vi "Replication and Deployment Utility.vi"() -> ()   [LabVIEW 2016]
uses:
  subVIs/TypeDefs/rad_State Data.ctl
  subVIs/Targets/TypeDefs/rad_Targets Settings.ctl
  subVIs/Targets/TypeDefs/rad_Target Information.ctl
  subVIs/Targets/TypeDefs/rad_Target Network Settings.ctl
  subVIs/App Images/TypeDefs/rad_App Images Settings.ctl
  subVIs/App Images/TypeDefs/rad_AppImage Information.ctl
  subVIs/App Images/TypeDefs/rad_Application Image Properties.ctl
  subVIs/App Images/TypeDefs/rad_FPGA Properties.ctl
  subVIs/App Images/TypeDefs/rad_FPGA Flash Properties.ctl
  subVIs/Util/Controls/Exit Button.ctl
  subVIs/Util/Controls/Retrieve Button.ctl
  subVIs/Util/Controls/Refresh Button.ctl
  subVIs/Util/Controls/Configure Button.ctl
  subVIs/Util/Controls/Deploy Button.ctl
  subVIs/Util/Controls/Select All Button.ctl
  subVIs/Util/Controls/Add Target Button.ctl
  subVIs/Util/Controls/Compare Button.ctl
  subVIs/Util/FP Control/FP Control Functions.ctl
  <vilib>/Utility/miscctls.llb/LVRowAndColumnUnsignedTypeDef.ctl
  subVIs/RT Image Compare/TypeDefs/rad_Comparison Modes.ctl
  <vilib>/nisyscfg/Close (System).vi
  subVIs/rad_Globals.vi
  <vilib>/nisyscfg/nisyscfg.lvlib
  <resource>/objmgr/nisysapi.rc
panel:
  in  "Targets Settings":bool
  in  "Refresh Targets":T1
  in  "Target List":i32[](listbox)=[0]
  in  "Add Target":T2
  in  "Select All":T3
  in  "Configure Targets":T4
  in  "Compare":T5
  in  "Deploy":T6
  in  "Retrieve":T7
  in  "State":T8 {"Targets Information"."Primary NIC"."IP Address Request Mode" items=["Static"=1, "DHCP/Link-Local"=2, "Link-Local Only"=4, "DHCP Only"=8]}
  in  "App Images Settings":bool
  in  "Refresh Apps":T1
  in  "Exit":T17
  in  "App Images List":i32(listbox)=6
  in  "Configure App":T4
  # "Deployment Targets"
  # "Application Images"
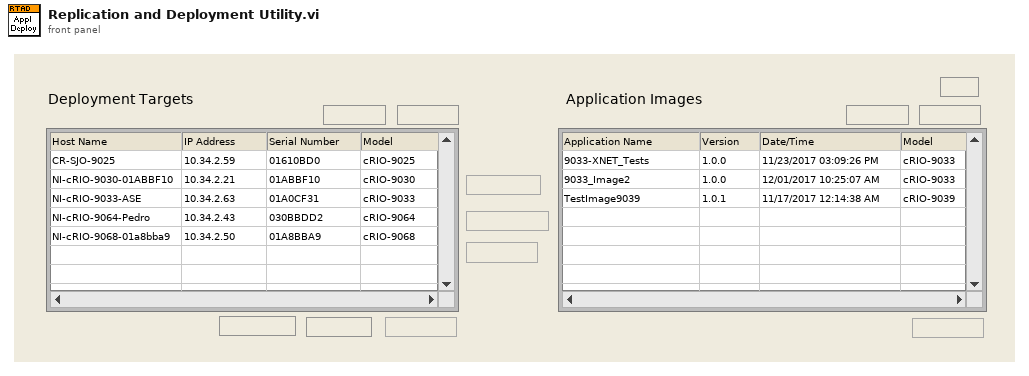
[diagram p1: front panel]
types:
  T1 = typedef "Refresh Button.ctl" = bool
  T2 = typedef "Add Target Button.ctl" = bool
  T3 = typedef "Select All Button.ctl" = bool
  T4 = typedef "Configure Button.ctl" = bool
  T5 = typedef "Compare Button.ctl" = bool
  T6 = typedef "Deploy Button.ctl" = bool
  T7 = typedef "Retrieve Button.ctl" = bool
  T8 = typedef "rad_State Data.ctl" = cluster{"Targets Settings":T9, "Targets Information":T10[], "App Images Settings":T12, "App Images Information":T13[], "Filtered Targets":i32[], "AppMode":string, "Configuration File Path":path, "Permissions":cluster{"Retrieve AppImgs":bool}, "User Added Targets":string[]}
  T9 = typedef "rad_Targets Settings.ctl" = cluster{"Target Types":string[], "Reduce Discovery Timeout":bool}
  T10 = typedef "rad_Target Information.ctl" = cluster{"Hostname":string, "Serial number":string, "Product name":string, "Product code":i32, "System status":string, "Credential type":enum16{"None/Unlocked", "FTP Password", "NIAuth Credentials"}, "User added?":bool, "Primary NIC":T11}
  T11 = typedef "rad_Target Network Settings.ctl" = cluster{"MAC address":string, "IP Address Request Mode":i32, "IP address":string, "Subnet mask":string, "Gateway":string, "DNS server":string}
  T12 = typedef "rad_App Images Settings.ctl" = cluster{"App Images Folder":path, "App Images Temp Folder":path, "CurrentVersion":string}
  T13 = typedef "rad_AppImage Information.ctl" = cluster{"AppImage Properties":T14, "AppImage Path":path}
  T14 = typedef "rad_Application Image Properties.ctl" = cluster{"Name":string, "Version":string, "Time":timestamp, "Description":string, "Key":string, "Chassis":string, "FPGA Properties":T15, "Model":string, "Retrieve":string[], "Deploy":string[], "Installed Software":string[]}
  T15 = typedef "rad_FPGA Properties.ctl" = T16[]
  T16 = typedef "rad_FPGA Flash Properties.ctl" = cluster{"Resource Name":string, "Path":path}
  T17 = typedef "Exit Button.ctl" = bool
  T18 = typedef "LVPoint32TypeDef.ctl" = cluster{"Horizontal":i32, "Vertical":i32}
  T19 = typedef "LVRowAndColumnTypeDef.ctl" = cluster{"Row":i32, "Column":i32}
  T20 = typedef "FP Control Functions.ctl" = enum16{"Open", "Close", "Bring To Front", "Center"}
  T21 = typedef "LVRowAndColumnUnsignedTypeDef.ctl" = cluster{"Row":u32, "Column":u32}
  T22 = typedef "rad_Comparison Modes.ctl" = enum32{"Compare Local Image With Controller", "Compare Two Local Images"}
  T23 = enum8{"Enabled", "Disabled", "Disabled and Grayed Out"}
  T24 = enum32{"invalid app kind", "Development System", "Run Time System", "Student Edition", "Embedded LabVIEW", "Evaluation", "Custom"}
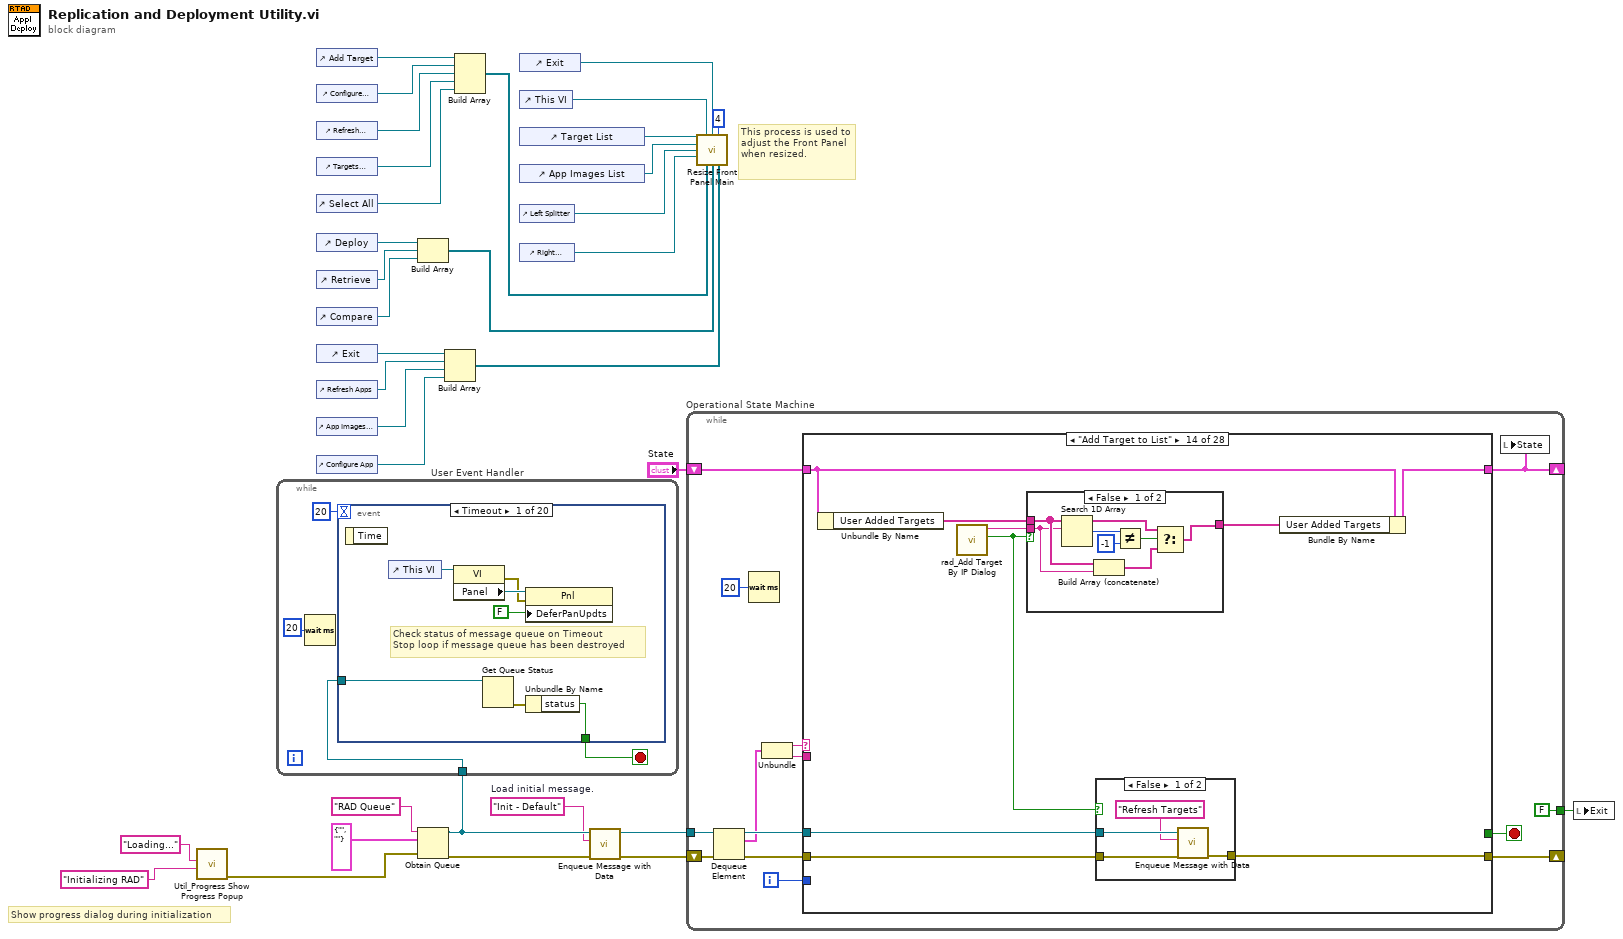
[diagram p0: block diagram]
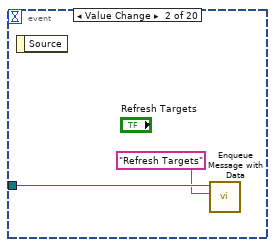
[diagram p2: hidden frame]
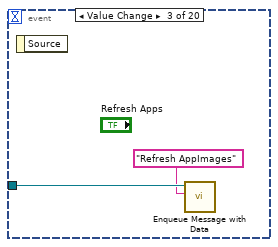
[diagram p3: hidden frame]
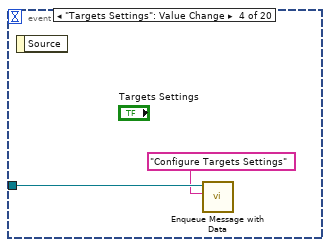
[diagram p4: hidden frame]
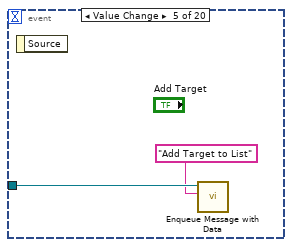
[diagram p5: hidden frame]
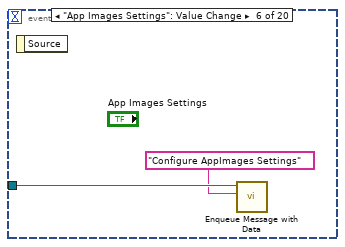
[diagram p6: hidden frame]
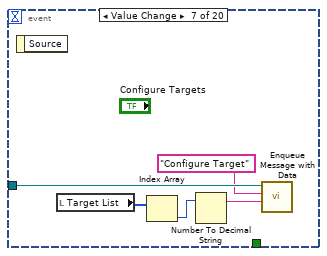
[diagram p7: hidden frame]
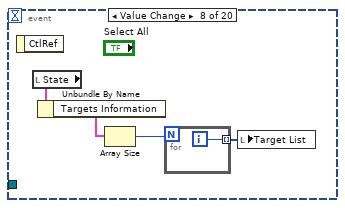
[diagram p8: hidden frame]
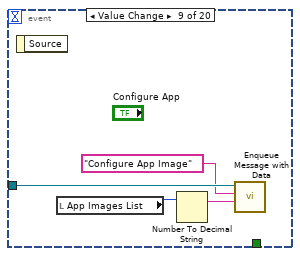
[diagram p9: hidden frame]
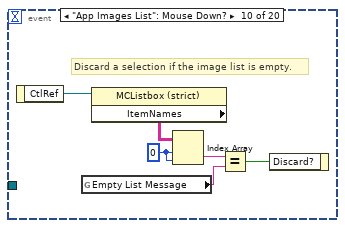
[diagram p10: hidden frame]
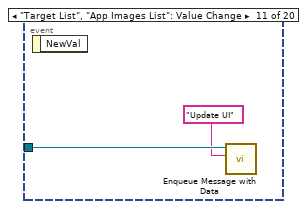
[diagram p11: hidden frame]
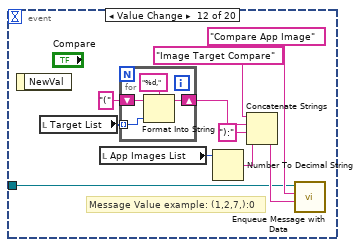
[diagram p12: hidden frame]
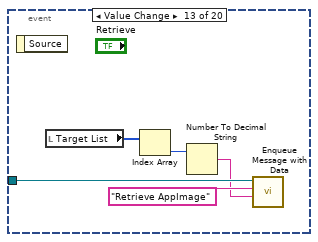
[diagram p13: hidden frame]
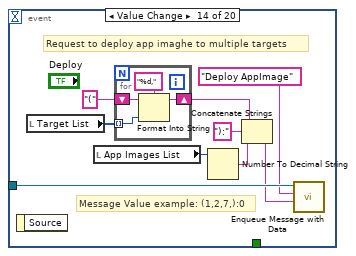
[diagram p14: hidden frame]
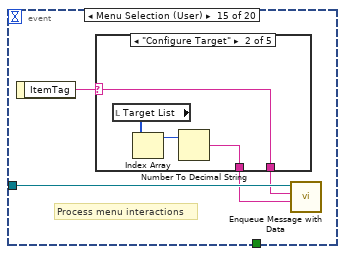
[diagram p15: hidden frame]
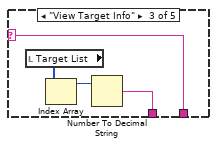
[diagram p17: hidden frame]
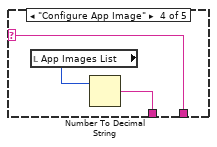
[diagram p18: hidden frame]
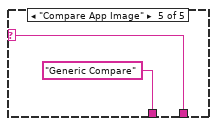
[diagram p19: hidden frame]
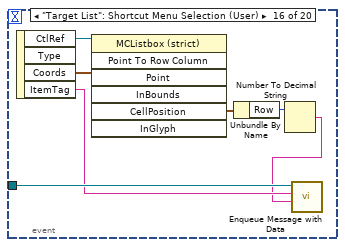
[diagram p20: hidden frame]
diagram:
  w4 = "Init - Default"  # Load initial message.
  # "Show progress dialog during initialization"
  # "This process is used to adjust the Front Panel when resized."
  n1 = call "Util_Progress Show Progress Popup.vi"("Title"="Initializing RAD", "Message"="Loading...") -> ("error out"=w1:errorcluster)  [unwired: 2 in, 7 out]
  n2 = control-ref of="Add Target"() -> (w25:refnum<vi>)
  n3 = control-ref of="Configure Targets"() -> (w24:refnum<vi>)
  n4 = control-ref of="Refresh Targets"() -> (w23:refnum<vi>)
  n5 = control-ref of="Targets Settings"() -> (w22:refnum<vi>)
  n6 = control-ref of="Select All"() -> (w21:refnum<vi>)
  n7 = control-ref of="Deploy"() -> (w19:refnum<vi>)
  n8 = control-ref of="Retrieve"() -> (w18:refnum<vi>)
  n9 = control-ref of="Compare"() -> (w17:refnum<vi>)
  n10 = control-ref of="Exit"() -> (w15:refnum<vi>)
  n11 = control-ref of="Refresh Apps"() -> (w14:refnum<vi>)
  n12 = control-ref of="App Images Settings"() -> (w13:refnum<vi>)
  n13 = control-ref of="Configure App"() -> (w12:refnum<vi>)
  n14 = Build Array(w19, w18, w17) -> (w16:refnum<vi>[])
  n15 = Obtain Queue(name (unnamed)="RAD Queue" ("message queue name"), element data type=cluster{string, string} {"", ""}, error in (no error)=w1) -> (queue out=w9:refnum<queue>, error out=w7:errorcluster)  [unwired: 2 in, 1 out]
  n16 = while "User Event Handler" {
    tunnel: w9 -> [w36]
    stop <- w37 stop-if-true
    n17 = Wait (ms)(milliseconds to wait=u32 20) -> ()  [unwired: 1 out]
    n18 = event shown="[0] Timeout" {
      selector: _ -> [_ _ _ _ _ _ _ _ _ _ _ _ _ _ _ _ _ _ _ _]
      dyn-events: _ -> [_ _ _ _ _ _ _ _ _ _ _ _ _ _ _ _ _ _ _ _]
      timeout: 20 -> [_ _ _ _ _ _ _ _ _ _ _ _ _ _ _ _ _ _ _ _]
      tunnel: [w43 _ _ _ _ _ _ _ _ _ _ _ _ _ _ _ _ _ TRUE ("Discard?") w159] -> w37
      tunnel: w36 -> [w45 w47 w49 w51 w53 w55 w58 _ w68 _ w77 w80 w94 w99 w112 w130 _ w149 w155 w158]
      event Timeout {
        # "Check status of message queue on Timeout\nStop loop if message queue has been destroyed"
        n19 = event-data() -> ()  [unwired: 2 out]
        n20 = control-ref of="This VI"() -> (w39:refnum<vi>)
        n21 = property class="VI"(reference=w39) -> (error out=w40:errorcluster, "Panel"=w42:refnum<vi>)  [unwired: 1 in, 1 out]
        n22 = Get Queue Status(queue=w45) -> (error out=w44:errorcluster)  [unwired: 1 in, 8 out]
        n23 = property class="Pnl"(reference=w42, error in=w40, "DeferPanUpdts"=FALSE ("Defer Panel Updates")) -> ()  [unwired: 2 out]
        n24 = Unbundle By Name(w44) -> ("status"=w43:bool)
      }
      event Value Change {
        n25 = event-data() -> ()  [unwired: 2 out]
        n26 = call "Enqueue Message with Data.vi"("message ID"="Refresh Targets", "queue in"=w47) -> ()  [unwired: 8 in, 2 out]
      }
      event Value Change {
        n27 = event-data() -> ()  [unwired: 2 out]
        n28 = call "Enqueue Message with Data.vi"("message ID"="Refresh AppImages", "queue in"=w49) -> ()  [unwired: 8 in, 2 out]
      }
      event "Targets Settings": Value Change {
        n29 = event-data() -> ()  [unwired: 2 out]
        n30 = call "Enqueue Message with Data.vi"("message ID"="Configure Targets Settings", "queue in"=w51) -> ()  [unwired: 8 in, 2 out]
      }
      event Value Change {
        n31 = event-data() -> ()  [unwired: 2 out]
        n32 = call "Enqueue Message with Data.vi"("message ID"="Add Target to List" ("Message Name"), "queue in"=w53) -> ()  [unwired: 8 in, 2 out]
      }
      event "App Images Settings": Value Change {
        n33 = event-data() -> ()  [unwired: 2 out]
        n34 = call "Enqueue Message with Data.vi"("message ID"="Configure AppImages Settings", "queue in"=w55) -> ()  [unwired: 8 in, 2 out]
      }
      event Value Change {
        n35 = event-data() -> ()  [unwired: 2 out]
        n36 = local read "Target List"() -> (w59:i32[])
        n37 = Index Array(array=w59) -> (element=w60:i32)  [unwired: 1 in]
        n38 = Number To Decimal String(number=w60) -> (decimal integer string=w56:string)  [unwired: 1 out]
        n39 = call "Enqueue Message with Data.vi"("extra data"=w56, "message ID"="Configure Target", "queue in"=w58) -> ()  [unwired: 7 in, 2 out]
      }
      event Value Change {
        n40 = event-data() -> ()  [unwired: 2 out]
        n41 = local read "State"() -> (w63:T8)
        n42 = Unbundle By Name(w63) -> ("Targets Information"=w62:T10[])
        n43 = Array Size(array=w62) -> (size(s)=w61:i32)
        n44 = for {
          N: w61 -> [_]
          tunnel: [w65] -> w64 mode=indexing
          i -> [w65]
        }
        n45 = local write "Target List"(w64) -> ()
      }
      event Value Change {
        n46 = event-data() -> ()  [unwired: 2 out]
        n47 = local read "App Images List"() -> (w69:i32)
        n48 = Number To Decimal String(number=w69) -> (decimal integer string=w66:string)  [unwired: 1 out]
        n49 = call "Enqueue Message with Data.vi"("extra data"=w66, "message ID"="Configure App Image", "queue in"=w68) -> ()  [unwired: 7 in, 2 out]
      }
      event "App Images List": Mouse Down? {
        w73 = 0 ("index (row)")
        # "Discard a selection if the image list is empty."
        n50 = event-data() -> ("CtlRef"=w75:refnum<vi>)  [unwired: 1 out]
        n51 = global read "rad_Globals.vi" "Empty List Message"() -> (w71:string)
        n52 = property class="MCListbox (strict)"(reference=w75) -> ("ItemNames"=w74:string[][])  [unwired: 1 in, 2 out]
        n53 = Index Array(array=w74, index (row)=w73, index (col)=w73) -> (element=w72:string)
        n54 = Equal?(x=w72, y=w71) -> (x = y?=w70:bool)
        n55 = event-data("Discard?"=w70) -> ()  [unwired: 1 in, 1 out]
      }
      event "Target List", "App Images List": Value Change {
        n56 = event-data() -> ()  [unwired: 2 out]
        n57 = call "Enqueue Message with Data.vi"("message ID"="Update UI" ("Message"), "queue in"=w77) -> ()  [unwired: 8 in, 2 out]
      }
      event Value Change {
        # "Message Value example: (1,2,7,):0"
        n58 = event-data() -> ()  [unwired: 2 out]
        n59 = local read "Target List"() -> (w84:i32[])
        n60 = local read "App Images List"() -> (w83:i32)
        n61 = for {
          shift-right: [w91] -> w85
          shift-left: "(" -> [w89]
          tunnel: w84 -> [w90] mode=indexing
          n62 = Format Into String(format string="%d,", initial string=w89, w90) -> (resulting string=w91:string)  [unwired: 1 in, 1 out]
        }
        n63 = Number To Decimal String(number=w83) -> (decimal integer string=w82:string)  [unwired: 1 out]
        n64 = Concatenate Strings("Image Target Compare" ("string"), w85, "):" ("string"), w82) -> (w87:string)
        n65 = call "Enqueue Message with Data.vi"("extra data"=w87, "message ID"="Compare App Image", "queue in"=w80) -> ()  [unwired: 7 in, 2 out]
      }
      event Value Change {
        n66 = event-data() -> ()  [unwired: 2 out]
        n67 = local read "Target List"() -> (w95:i32[])
        n68 = Index Array(array=w95) -> (element=w96:i32)  [unwired: 1 in]
        n69 = Number To Decimal String(number=w96) -> (decimal integer string=w92:string)  [unwired: 1 out]
        n70 = call "Enqueue Message with Data.vi"("extra data"=w92, "message ID"="Retrieve AppImage", "queue in"=w94) -> ()  [unwired: 7 in, 2 out]
      }
      event Value Change {
        # "Request to deploy app imaghe to multiple targets"
        # "Message Value example: (1,2,7,):0"
        n71 = event-data() -> ()  [unwired: 2 out]
        n72 = local read "Target List"() -> (w101:i32[])
        n73 = local read "App Images List"() -> (w103:i32)
        n74 = for {
          shift-right: [w109] -> w100
          shift-left: "(" -> [w107]
          tunnel: w101 -> [w108] mode=indexing
          n75 = Format Into String(format string="%d,", initial string=w107, w108) -> (resulting string=w109:string)  [unwired: 1 in, 1 out]
        }
        n76 = Number To Decimal String(number=w103) -> (decimal integer string=w104:string)  [unwired: 1 out]
        n77 = Concatenate Strings(w100, "):" ("string"), w104) -> (w97:string)
        n78 = call "Enqueue Message with Data.vi"("extra data"=w97, "message ID"="Deploy AppImage", "queue in"=w99) -> ()  [unwired: 7 in, 2 out]
      }
      event Menu Selection (User) {
        # "Process menu interactions"
        n79 = event-data() -> ("ItemTag"=w113:string)  [unwired: 1 out]
        n80 = case shown="\"Configure Target\"" w113 {
          selector: w113 -> [w114 w116 w120 w124 w126]
          tunnel: [w114 w116 w120 w124 w126] -> w111
          tunnel: [_ w115 w119 w123 "Generic Compare"] -> w110
          frame Default {
          }
          frame "Configure Target" {
            n81 = local read "Target List"() -> (w118:i32[])
            n82 = Index Array(array=w118) -> (element=w117:i32)  [unwired: 1 in]
            n83 = Number To Decimal String(number=w117) -> (decimal integer string=w115:string)  [unwired: 1 out]
          }
          frame "View Target Info" {
            n84 = local read "Target List"() -> (w122:i32[])
            n85 = Index Array(array=w122) -> (element=w121:i32)  [unwired: 1 in]
            n86 = Number To Decimal String(number=w121) -> (decimal integer string=w119:string)  [unwired: 1 out]
          }
          frame "Configure App Image" {
            n87 = local read "App Images List"() -> (w125:i32)
            n88 = Number To Decimal String(number=w125) -> (decimal integer string=w123:string)  [unwired: 1 out]
          }
          frame "Compare App Image" {
          }
        }
        n89 = call "Enqueue Message with Data.vi"("extra data"=w110, "message ID"=w111, "queue in"=w112) -> ()  [unwired: 7 in, 2 out]
      }
      event "Target List": Shortcut Menu Selection (User) {
        n90 = event-data() -> ("CtlRef"=w132:refnum<vi>, "Coords"=w131:T18, "ItemTag"=w129:string)  [unwired: 2 out]
        n91 = invoke class="MCListbox (strict)" method="Point To Row Column"(reference=w132, "Point"=w131) -> ("CellPosition"=w134:T19)  [unwired: 5 in, 6 out]
        n92 = Unbundle By Name(w134) -> ("Row"=w133:i32)
        n93 = Number To Decimal String(number=w133) -> (decimal integer string=w128:string)  [unwired: 1 out]
        n94 = call "Enqueue Message with Data.vi"("extra data"=w128, "message ID"=w129, "queue in"=w130) -> ()  [unwired: 7 in, 2 out]
      }
      event "App Images List": Shortcut Menu Activation? {
        n95 = event-data() -> ("MenuRef"=w136:refnum<k9>)  [unwired: 1 out]
        n96 = global read "rad_Globals.vi" "Manager Permissions"() -> (w135:bool)
        n97 = case shown="False" w135 {
          tunnel: w136 -> [w141 _]
          tunnel: [w138 _] -> _
          frame False {
            w137 = string[] ["View App Image Info"] ("item names")
            n98 = Delete Menu Items(9:w141) -> (0:w139:errorcluster, 3:w140:refnum<k9>)  [unwired: 3 in]
            n99 = Insert Menu Items(6:w139, 7:w137, 8:w137, 9:w140) -> (0:w138:errorcluster)  [unwired: 2 in, 2 out]
          }
          frame True {
          }
        }
        n100 = event-data() -> ()  [unwired: 2 in, 1 out]
      }
      event "App Images List": Shortcut Menu Selection (User) {
        n101 = event-data() -> ("CtlRef"=w151:refnum<vi>, "Coords"=w150:T18, "ItemTag"=w142:string)  [unwired: 1 out]
        n102 = Equal?(x=w142, y="Compare App Image") -> (x = y?=w147:bool)
        n103 = invoke class="MCListbox (strict)" method="Point To Row Column"(reference=w151, "Point"=w150) -> ("CellPosition"=w153:T19)  [unwired: 5 in, 6 out]
        n104 = Unbundle By Name(w153) -> ("Row"=w152:i32)
        n105 = Number To Decimal String(number=w152) -> (decimal integer string=w144:string)  [unwired: 1 out]
        n106 = Concatenate Strings("Only Image Selected(" ("string"), w144) -> (w146:string)
        n107 = Select(t=w146, s=w147, f=w144) -> (s? t:f=w143:string)
        n108 = call "Enqueue Message with Data.vi"("extra data"=w143, "message ID"=w142, "queue in"=w149) -> ()  [unwired: 7 in, 2 out]
      }
      event Value Change {
        n109 = event-data() -> ()  [unwired: 2 out]
        n110 = call "Enqueue Message with Data.vi"("message ID"="Exit", "queue in"=w155) -> ()  [unwired: 8 in, 2 out]
      }
      event Panel Close? {
        w159 = TRUE ("Discard?")
        # "Intercepts the upper right close panel\noperation to allow a smooth shutdown\nas opposed to immediately killing the app."
        n111 = event-data() -> ()  [unwired: 2 out]
        n112 = call "Enqueue Message with Data.vi"("message ID"="Exit", "queue in"=w158) -> ()  [unwired: 8 in, 2 out]
        n113 = event-data("Discard?"=w159) -> ()  [unwired: 1 in, 1 out]
      }
    }
  }
  n114 = Build Array(w15, w14, w13, w12) -> (w11:refnum<vi>[])
  n115 = Build Array(w25, w24, w23, w22, w21) -> (w20:refnum<vi>[])
  n116 = control-ref of="Exit"() -> (w31:refnum<vi>)
  n117 = control-ref of="This VI"() -> (w30:refnum<vi>)
  n118 = control-ref of="Target List"() -> (w29:refnum<vi>)
  n119 = control-ref of="App Images List"() -> (w28:refnum<vi>)
  n120 = control-ref of="Left Splitter"() -> (w27:refnum<vi>)
  n121 = control-ref of="Right Splitter"() -> (w26:refnum<vi>)
  n122 = call "Enqueue Message with Data.vi"("error in (no error)"=w7, "message ID"=w4, "queue in"=w9) -> ("error out"=w6:errorcluster, "queue out"=w8:refnum<queue>)  [unwired: 7 in]
  n123 = while "Operational State Machine" {
    shift-left: w6 -> [w165]
    shift-right: [w166] -> _
    tunnel: w8 -> [w170]
    shift-left: "State" -> [w173]
    shift-right: [w167] -> _
    tunnel: [T17 FALSE ("Exit")] -> w10
    i -> [w169]
    stop <- w163 stop-if-true
    n124 = Dequeue Element(queue=w170, error in (no error)=w165) -> (queue out=w172:refnum<queue>, element=w168:cluster{string, string}, error out=w171:errorcluster)  [unwired: 1 in, 1 out]
    n125 = Wait (ms)(milliseconds to wait=u32 20) -> ()  [unwired: 1 out]
    n126 = Unbundle(w168) -> (w162:string, w161:string)
    n127 = case shown="\"Add Target to List\"" w162 {
      tunnel: [w175 w177 w191 w219 w240 w261 w292 w307 w309 w313 w319 w331 w339 w355 w377 w393 w409 w422 w433 w435 w456 w471 w483 w491 w560 w575 w607 w623] -> w167
      tunnel: w173 -> [w175 w177 w195 w218 w241 w257 w292 w307 w309 w313 w319 w331 w340 w356 w378 w394 w409 w427 w433 w439 w457 w470 w483 w491 w560 w576 w607 w623]
      tunnel: w172 -> [_ _ w179 w202 _ w253 _ _ _ _ w326 _ w337 w351 w376 w392 _ w421 _ w437 w450 w473 _ _ w547 w579 w592 w624]
      tunnel: w171 -> [w174 w176 w184 w201 w239 w255 w289 w308 w310 w312 w325 w330 w336 w353 w372 w391 w402 w420 w432 w436 w452 w472 w484 w490 w549 w582 w595 w628]
      tunnel: w169 -> [_ _ _ _ _ _ _ _ _ _ _ _ _ _ _ _ _ _ _ _ _ _ _ _ _ _ _ _]
      tunnel: w161 -> [_ _ _ _ _ _ _ _ _ _ _ _ _ _ w386 _ w407 w431 _ _ w460 _ w480 w487 w558 w584 w606 _]
      tunnel: [w174 w176 w178 w203 w239 w254 w273 w308 w310 errorcluster {"status"=FALSE, "code"=0, "source"=""} ("error out") w320 w330 w338 w352 w374 w388 w402 w419 w432 w438 w451 w467 w484 w485 w548 w580 w594 w625] -> w166
      tunnel: [_ _ _ _ _ _ _ _ _ _ TRUE _ _ _ _ _ _ _ _ _ _ _ _ _ _ _ _ _] -> w163
      frame "Missing Message Handler", Default {
      }
      frame "**** General Application Messages ****" {
      }
      frame "Init - Default" {
        w185 = T21 {"Row"=0, "Column"=0} ("Top Left Visible Cell")
        w187 = string[][] [] ("Item Names")
        w194 = u8 2 ("Disabled")
        # "Initialize the UI"
        # "Application Folder"
        # "Default AppImages folder"
        n128 = call "Util_App Application Directory.vi"() -> ("Application Directory"=w190:path)  [unwired: 11 out]
        n129 = call "Enqueue Message with Data.vi"("error in (no error)"=w184, "message ID"="Init - Load Config", "queue in"=w179) -> ("error out"=w183:errorcluster, "queue out"=w182:refnum<queue>)  [unwired: 7 in]
        n130 = local write "App Images List"(-1 ("App Images List")) -> ()
        n131 = local write "Target List"(i32[] [] ("Target List")) -> ()
        n132 = Build Path(base path=w190, name or relative path="appimages") -> (appended path=w196:path)
        n133 = Build Path(base path=w190, name or relative path="rad_config.ini" ("Config File Name")) -> (appended path=w188:path)
        n134 = call "Enqueue Message with Data.vi"("error in (no error)"=w183, "message ID"="Init - Configure Settings", "queue in"=w182) -> ("error out"=w178:errorcluster)  [unwired: 7 in, 1 out]
        n135 = property on="Configure App" class="Bool"("Disabled"=w194) -> ()  [unwired: 2 in, 2 out]
        n136 = property on="Configure Targets" class="Bool"("Disabled"=w194) -> ()  [unwired: 2 in, 2 out]
        n137 = Bundle By Name(cluster=w195, "App Images Settings.App Images Folder"=w196, "Configuration File Path"=w188) -> (w191:T8)
        n138 = property on="Target List" class="MCListbox (strict)"("ItemNames"=w187, "TopLeft"=w185) -> ()  [unwired: 2 in, 2 out]
        n139 = property on="App Images List" class="MCListbox (strict)"("ItemNames"=w187, "TopLeft"=w185) -> ()  [unwired: 2 in, 2 out]
        n140 = call "Util_FP Control.vi"("Function"=FP_Control_Functions."Center") -> ()  [unwired: 10 in, 1 out]
      }
      frame "Init - Load Config" {
        # "Close Init\nDialog"
        n141 = call "rad_Load Config.vi"("error in (no error"=w201, "State in"=w218) -> ("error out"=w199:errorcluster, "State out"=w219:T8)  [unwired: 1 in, 7 out]
        n142 = call <vilib>:"Initialize Session.vi"("error in (no error)"=w199) -> ("error out"=w206:errorcluster, "Session out"=w207:refnum<k21>)  [unwired: 9 in]
        n143 = property class="System Session"(reference=w207, error in=w206) -> (reference out=w208:refnum<k21>, error out=w205:errorcluster, "InstalledVer"=w204:string)
        n144 = Scan From String(format string="%d.%d.%d", input string=w204) -> (output 1=w216:i32, output 2=w213:i32, output 3=w210:i32)  [unwired: 5 in, 3 out]
        n145 = call-poly <vilib>:"Close.vi"("error in (no error)"=w205, "Session in"=w208) -> ("error out"=w198:errorcluster)  [unwired: 9 in]
        n146 = Multiply(x=10, y=w213) -> (x*y=w211:i32)
        n147 = Multiply(x=100, y=w216) -> (x*y=w212:i32)
        n148 = call "Util_Progress Close Progress Popup.vi"("error in (no error)"=w198) -> ()  [unwired: 2 in, 9 out]
        n149 = Compound Arithmetic op=ADD(w212, w211, w210) -> (w209:i32)
        n150 = case shown="Default" w209 {
          tunnel: [w230 TRUE ("T button?")] -> w200
          frame Default {
            n151 = Two Button Dialog(message="RAD requires newer functionality\nthan the software you have installed.\nPlease update to NI System Configuration\nversion 14.0 or higher.", 1:"Exit" ("F button name (\"Cancel\")"), 2:"Continue" ("T button name (\"OK\")")) -> (T button?=w230:bool)
          }
          frame 1400.. {
            # "RAD 14.0 has been fully tested\nwith NI System Configuration 14.0.\nFuture versions should work fine too."
          }
        }
        n152 = case shown="True" w200 {
          tunnel: w199 -> [w221 w228]
          tunnel: [w222 w223] -> w203
          tunnel: w202 -> [_ w227]
          frame False {
            n153 = property on="Exit" class="Bool (strict)"(error in=w221, "Val(Sgnl)"=T17 TRUE ("Value (Signaling)")) -> (error out=w222:errorcluster)  [unwired: 1 in, 1 out]
          }
          frame True {
            n154 = call "Enqueue Message with Data.vi"("error in (no error)"=w228, "message ID"="Refresh Targets", "queue in"=w227) -> ("error out"=w224:errorcluster, "queue out"=w225:refnum<queue>)  [unwired: 7 in]
            n155 = call "Enqueue Message with Data.vi"("error in (no error)"=w224, "message ID"="Refresh AppImages", "queue in"=w225) -> ("error out"=w223:errorcluster)  [unwired: 7 in, 1 out]
          }
        }
      }
      frame "Init - Configure Settings" {
        # "The temp folder should always be writable."
        # "Set permissions and update UI based on application\nmode. Disable or hide controls not appropriate\nfor current application mode."
        # "Apply configuration settings from config file"
        n156 = Unbundle By Name(w241) -> ("AppMode"=w242:string)
        n157 = case shown="\"Manager\"" w242 {
          tunnel: [TRUE ("Visible") FALSE ("Visible")] -> w238
          frame "Manager" {
          }
          frame Default {
          }
        }
        n158 = call <vilib>:"Generate Temporary File Path.vi"("Temporary File Extension (tmp)"="rad") -> ("Unique Temporary File Path"=w235:path)  [unwired: 9 in, 1 out]
        n159 = property on="Retrieve" class="Bool"("Visible"=w238) -> ()  [unwired: 2 in, 2 out]
        n160 = property on="Configure App" class="Bool"("Visible"=w238) -> ()  [unwired: 2 in, 2 out]
        n161 = Bundle By Name(cluster=w241, "App Images Settings.App Images Temp Folder"=w235, "Permissions.Retrieve AppImgs"=w238) -> (w240:T8)
        n162 = global write "rad_Globals.vi" "Manager Permissions"(w238) -> ()
        n163 = global write "rad_Globals.vi" "ShownImageVersionDialog"(FALSE ("ShownNewerVersionDialog")) -> ()
      }
      frame "Update UI" {
        # "Scroll the lists to the top if no item is selected."
        # "Display target and app images based on settings\nfor each of these tables"
        n164 = Unbundle By Name(w257) -> ("Targets Information"=w264:T10[], "Targets Settings.Target Types"=w256:string[], "App Images Information"=w258:T13[])
        n165 = call "rad_Format Application Images Information.vi"("App Images Information"=w258) -> ("App Images Information"=w259:string[][])  [unwired: 10 out]
        n166 = call "rad_FilterTargets.vi"("Target Types"=w256, "Targets Information"=w264) -> ("Filtered Targets"=w262:i32[], "Targets Information"=w263:T10[])  [unwired: 8 out]
        n167 = Bundle By Name(cluster=w257, "Filtered Targets"=w262) -> (w261:T8)
        n168 = call "rad_Format Target Information.vi"("Targets Information"=w263) -> ("Targets Information"=w260:string[][])  [unwired: 10 out]
        n169 = property on="App Images List" class="MCListbox (strict)"("ItemNames"=w259) -> (error out=w250:errorcluster)  [unwired: 2 in, 1 out]
        n170 = property on="Target List" class="MCListbox (strict)"("ItemNames"=w260) -> (error out=w251:errorcluster)  [unwired: 2 in, 1 out]
        n171 = flat-sequence {
          tunnel: w251 -> [_]
          tunnel: w250 -> [_]
          tunnel: ["App Images List"] -> w248
          tunnel: [w268] -> w249
          tunnel: [-1 ("y")] -> w246
          frame #0 {
            n172 = Array Size(array="Target List") -> (size(s)=w268:i32)
          }
        }
        n173 = Equal?(x=w248, y=w246) -> (x = y?=w245:bool)
        n174 = Equal To 0?(x=w249) -> (x = 0?=w247:bool)
        n175 = call "Enqueue Message with Data.vi"("error in (no error)"=w255, "message ID"="Update Buttons and Menus" ("Message Name"), "queue in"=w253) -> ("error out"=w254:errorcluster)  [unwired: 7 in, 1 out]
        n176 = case shown="True" w245 {
          frame False {
          }
          frame True {
            n177 = property on="App Images List" class="MCListbox (strict)"("TopLeft"=T21 {"Row"=0, "Column"=0} ("Top Left Visible Cell")) -> ()  [unwired: 2 in, 2 out]
          }
        }
        n178 = case shown="True" w247 {
          frame False {
          }
          frame True {
            n179 = property on="Target List" class="MCListbox (strict)"("TopLeft"=T21 {"Row"=0, "Column"=0} ("Top Left Visible Cell")) -> ()  [unwired: 2 in, 2 out]
          }
        }
      }
      frame "Update Buttons and Menus" {
        w277 = T23."Disabled and Grayed Out" ("Disabled")
        w278 = T23."Enabled" ("Disabled")
        # "Enable and disable buttons and \nenu items based on selections\nin both tables"
        n180 = local read "App Images List"() -> (w290:i32)
        n181 = local read "Target List"() -> (w291:i32[])
        n182 = Unbundle By Name(w292) -> ("Permissions.Retrieve AppImgs"=w271:bool)
        n183 = call "rad_Button and Menu Status.vi"("Manager Permissions"=w271, "App Image List"=w290, "Target List"=w291) -> ("Retrieve AppImage"=w281:bool, "Deploy AppImage"=w283:bool, "View Target Info"=w288:bool, "Configure App Image"=w285:bool, "Compare"=w279:bool, "Configure Target"=w287:bool)  [unwired: 3 in]
        n184 = Current VI's Menubar() -> (w293:refnum<k9>)
        n185 = Set Menu Item Info(7:"Configure Target" ("item tag"), 8:w289, 9:w287, 11:w293) -> (0:w295:errorcluster, 3:w297:refnum<k9>)  [unwired: 3 out]
        n186 = Select(t=w278, s=w287, f=w277) -> (s? t:f=w286:T23)
        n187 = Select(t=w278, s=w285, f=w277) -> (s? t:f=w284:T23)
        n188 = Select(t=w278, s=w283, f=w277) -> (s? t:f=w282:T23)
        n189 = Select(t=w278, s=w281, f=w277) -> (s? t:f=w280:T23)
        n190 = Select(t=w278, s=w279, f=w277) -> (s? t:f=w276:T23)
        n191 = Set Menu Item Info(7:"Configure App Image" ("item tag"), 8:w295, 9:w285, 11:w297) -> (0:w298:errorcluster, 3:w299:refnum<k9>)  [unwired: 3 out]
        n192 = Set Menu Item Info(7:"View Target Info" ("item tag"), 8:w298, 9:w288, 11:w299) -> (0:w300:errorcluster, 3:w301:refnum<k9>)  [unwired: 3 out]
        n193 = Set Menu Item Info(7:"Deploy AppImage" ("item tag"), 8:w300, 9:w283, 11:w301) -> (0:w302:errorcluster, 3:w303:refnum<k9>)  [unwired: 3 out]
        n194 = property on="Configure Targets" class="Bool"("Disabled"=w286) -> ()  [unwired: 2 in, 2 out]
        n195 = property on="Configure App" class="Bool"("Disabled"=w284) -> ()  [unwired: 2 in, 2 out]
        n196 = property on="Deploy" class="Bool"("Disabled"=w282) -> ()  [unwired: 2 in, 2 out]
        n197 = property on="Retrieve" class="Bool"("Disabled"=w280) -> ()  [unwired: 2 in, 2 out]
        n198 = property on="Compare" class="Bool"("DisabledEnum"=w276) -> ()  [unwired: 2 in, 2 out]
        n199 = Set Menu Item Info(7:"Retrieve AppImage" ("item tag"), 8:w302, 9:w281, 11:w303) -> (0:w274:errorcluster, 3:w275:refnum<k9>)  [unwired: 3 out]
        n200 = Set Menu Item Info(7:"Convert Images" ("item tag"), 8:w274, 9:w271, 11:w275) -> (0:w273:errorcluster)  [unwired: 4 out]
      }
      frame "Status" {
      }
      frame "About" {
        # "Show About dialog"
        n201 = call "rad_About Dialog.vi"() -> ()  [unwired: 12 out]
      }
      frame "Error" {
        # "Display run-time error message\nAdd code to log error if desired"
        n202 = disable-structure shown="TARGET_TYPE==Windows" {
          disable-tunnel: w312 -> [w314 _]
          frame condition #0 (active) {
            n203 = call <vilib>:"Simple Error Handler.vi"("error in (no error)"=w314) -> ()  [unwired: 1 in, 8 out]
          }
          frame condition #1 {
          }
        }
      }
      frame "Exit" {
        # "Store current settings in the application config file"
        # "Close the front panel if the application is running as an EXE"
        n204 = Release Queue(queue=w326, force destroy? (F)=TRUE, error in (no error)=w325) -> (error out=w318:errorcluster)  [unwired: 2 out]
        n205 = Open Application Reference() -> (0:w323:errorcluster, 3:w324:refnum<vi>)  [unwired: 4 in]
        n206 = call "rad_Save Config.vi"("error in (no error"=w318, "State"=w319) -> ("error out"=w317:errorcluster)  [unwired: 1 in, 8 out]
        n207 = property class="App"(reference=w324, error in=w323) -> ("App.Kind"=w322:T24)  [unwired: 2 out]
        n208 = case shown="\"Run Time System\"" w322 {
          frame Default {
          }
          frame "Run Time System" {
            # "Close FP in EXE"
            n209 = Current VI's Path() -> (path=w329:path)
            n210 = Open VI Reference(vi path=w329) -> (vi reference=w328:refnum<vi>, error out=w327:errorcluster)  [unwired: 5 in]
            n211 = invoke class="VI" method="FP.Close"(reference=w328, error in=w327) -> ()  [unwired: 1 in, 3 out]
          }
        }
        n212 = property on="Exit" class="Bool (strict)"(error in=w317, "Val(Sgnl)"=TRUE) -> (error out=w320:errorcluster)  [unwired: 1 in, 1 out]
      }
      frame "**** Target Messages ****" {
      }
      frame "Refresh Targets" {
        # "Refresh list of RT targets on the local subnet.\nShow progress dialog during this process."
        n213 = Unbundle By Name(w340) -> ("Targets Settings.Reduce Discovery Timeout"=w333:bool, "User Added Targets"=w346:string[], "Targets Settings.Target Types"=w332:string[])
        n214 = call "Util_Progress Show Progress Popup.vi"("error in (no error)"=w336, "Title"="Discovering Targets", "Message"="Refreshing target list...") -> ("error out"=w334:errorcluster)  [unwired: 1 in, 7 out]
        n215 = Search 1D Array(1D array=w332, element="User Targets Only") -> (index of element=w343:i32)  [unwired: 1 in]
        n216 = Not Equal?(x=w343, y=-1) -> (x != y?=w341:bool)
        n217 = call "rad_Refresh Target Information.vi"("Reduce Discovery Timeout"=w333, "error in (no error)"=w334, "User Added Targets Only"=w341, "User Added Targets"=w346) -> ("error out"=w335:errorcluster, "Targets Information"=w345:T10[])  [unwired: 6 in]
        n218 = call "Util_Progress Close Progress Popup.vi"("error in (no error)"=w335) -> ()  [unwired: 2 in, 9 out]
        n219 = Bundle By Name(cluster=w340, "Targets Information"=w345) -> (w339:T8)
        n220 = call "Enqueue Message with Data.vi"("error in (no error)"=w335, "message ID"="Update UI", "queue in"=w337) -> ("error out"=w338:errorcluster)  [unwired: 7 in, 1 out]
      }
      frame "Add Target to List" {
        n221 = Unbundle By Name(w356) -> ("User Added Targets"=w358:string[])
        n222 = call "rad_Add Target By IP Dialog.vi"() -> ("Canceled?"=w350:bool, "IP Address"=w357:string)  [unwired: 10 in]
        n223 = case shown="False" w350 {
          tunnel: w358 -> [w366 w371]
          tunnel: w357 -> [w365 _]
          tunnel: [w367 w371] -> w354
          frame False {
            n224 = Search 1D Array(1D array=w366, element=w365) -> (index of element=w370:i32)  [unwired: 1 in]
            n225 = Build Array (concatenate)(w366, w365) -> (w364:string[])
            n226 = Not Equal?(x=w370, y=-1) -> (x != y?=w368:bool)
            n227 = Select(t=w366, s=w368, f=w364) -> (s? t:f=w367:string[])
          }
          frame True {
          }
        }
        n228 = case shown="False" w350 {
          tunnel: w353 -> [w362 w363]
          tunnel: [w361 w363] -> w352
          tunnel: w351 -> [w360 _]
          frame False {
            n229 = call "Enqueue Message with Data.vi"("error in (no error)"=w362, "message ID"="Refresh Targets" ("Message Name"), "queue in"=w360) -> ("error out"=w361:errorcluster)  [unwired: 7 in, 1 out]
          }
          frame True {
          }
        }
        n230 = Bundle By Name(cluster=w356, "User Added Targets"=w354) -> (w355:T8)
      }
      frame "Configure Target" {
        # "Update network settings/configuration of the selected RT target"
        n231 = Unbundle By Name(w378) -> ("Targets Information"=w382:T10[], "Filtered Targets"=w385:i32[])
        n232 = Decimal String To Number(string=w386) -> (number=w384:i32)  [unwired: 3 out]
        n233 = Index Array(array=w385, index=w384) -> (element=w380:i32)
        n234 = Index Array(array=w382, index=w380) -> (element=w383:T10)
        n235 = call "rad_Configure Target Dialog.vi"("Error In"=w372, "Target Information in"=w383) -> ("Error Out"=w373:errorcluster, "Target Information out"=w381:T10)  [unwired: 8 out]
        n236 = Replace Array Subset(array=w382, new element=w381, index=w380) -> (w379:T10[])
        n237 = call <vilib>:"General Error Handler.vi"("error in (no error)"=w373) -> ()  [unwired: 10 in, 5 out]
        n238 = Bundle By Name(cluster=w378, "Targets Information"=w379) -> (w377:T8)
        n239 = call "Enqueue Message with Data.vi"("error in (no error)"=w372, "message ID"="Update UI", "queue in"=w376) -> ("error out"=w374:errorcluster)  [unwired: 7 in, 1 out]
      }
      frame "Configure Targets Settings" {
        # "Update the RT Target settings >> select which types of RT targets to display in the table\nCompactRIO, PXI, FieldPoint, or Other"
        n240 = Unbundle By Name(w394) -> ("Targets Settings"=w389:T9)
        n241 = call "rad_Configure Targets Settings Dialog.vi"("Targets Settings"=w389) -> ("Targets Settings"=w390:T9)  [unwired: 10 out]
        n242 = Equal?(x=w390, y=w389) -> (x = y?=w387:bool)
        n243 = Bundle By Name(cluster=w394, "Targets Settings"=w390) -> (w393:T8)
        n244 = case shown="False" w387 {
          tunnel: w392 -> [w398 _]
          tunnel: w391 -> [w397 w399]
          tunnel: [w396 w399] -> w388
          frame False {
            n245 = call "Enqueue Message with Data.vi"("error in (no error)"=w397, "message ID"="Update UI", "queue in"=w398) -> ("error out"=w396:errorcluster)  [unwired: 7 in, 1 out]
          }
          frame True {
          }
        }
      }
      frame "View Target Info" {
        # "Display additional information about the selected RT target in a popup window"
        n246 = Unbundle By Name(w409) -> ("Targets Information"=w408:T10[], "Filtered Targets"=w406:i32[])
        n247 = Decimal String To Number(string=w407) -> (number=w405:i32)  [unwired: 3 out]
        n248 = Index Array(array=w406, index=w405) -> (element=w404:i32)
        n249 = Index Array(array=w408, index=w404) -> (element=w400:T10)
        n250 = call "rad_Get Target Info (IP).vi"("error in (no error)"=w402, "Target settings in"=w400) -> ("error out"=w401:errorcluster, "Target settings out"=w403:T10)  [unwired: 8 in]
        n251 = case shown="No Error" w401 {
          selector: w401 -> [_ w411]
          tunnel: w403 -> [w410 _]
          frame No Error {
            n252 = call "rad_Target Info Dialog.vi"("Target Information"=w410) -> ()  [unwired: 11 out]
          }
          frame Error {
            n253 = call <vilib>:"General Error Handler.vi"("error in (no error)"=w411) -> ()  [unwired: 10 in, 5 out]
          }
        }
      }
      frame "Delete Target" {
        n254 = Unbundle By Name(w427) -> ("Targets Information"=w426:T10[], "Filtered Targets"=w414:i32[], "User Added Targets"=w415:string[])
        n255 = Decimal String To Number(string=w431) -> (number=w417:i32)  [unwired: 2 in, 1 out]
        n256 = Index Array(array=w414, index=w417) -> (element=w416:i32)
        n257 = Delete From Array(array=w426, length=1, index=w416) -> (deleted portion=w424:T10[], array with subset deleted=w425:T10[])
        n258 = Index Array(array=w424) -> (element=w423:T10)  [unwired: 1 in]
        n259 = Unbundle By Name(w423) -> ("Primary NIC.IP address"=w413:string)
        n260 = Search 1D Array(1D array=w415, element=w413) -> (index of element=w430:i32)  [unwired: 1 in]
        n261 = call "Enqueue Message with Data.vi"("error in (no error)"=w420, "message ID"="Update UI" ("Message Name"), "queue in"=w421) -> ("error out"=w419:errorcluster)  [unwired: 7 in, 1 out]
        n262 = Delete From Array(array=w415, length=1, index=w430) -> (array with subset deleted=w412:string[])  [unwired: 1 out]
        n263 = Bundle By Name(cluster=w427, "Targets Information"=w425, "User Added Targets"=w412) -> (w422:T8)
      }
      frame "**** Image Messages ****" {
      }
      frame "Refresh AppImages" {
        # "Update list of application images available in the configured folder"
        n264 = Unbundle By Name(w439) -> ("App Images Settings.App Images Temp Folder"=w440:path, "App Images Settings.App Images Folder"=w444:path)
        n265 = call "Util_Progress Show Progress Popup.vi"("Title"="Refreshing App Images", "Message"="Refreshing application images list...") -> ("error out"=w443:errorcluster)  [unwired: 2 in, 7 out]
        n266 = call "rad_List Application Images.vi"("App Image Temp Folder"=w440, "error in (no error)"=w443, "App Images Folder"=w444) -> ("error out"=w442:errorcluster, "Application Images Infomration"=w441:T13[])  [unwired: 1 in, 6 out]
        n267 = Bundle By Name(cluster=w439, "App Images Information"=w441) -> (w435:T8)
        n268 = call "Util_Progress Close Progress Popup.vi"("error in (no error)"=w442) -> ()  [unwired: 2 in, 9 out]
        n269 = call "Enqueue Message with Data.vi"("error in (no error)"=w436, "message ID"="Update UI" ("Message"), "queue in"=w437) -> ("error out"=w438:errorcluster)  [unwired: 7 in, 1 out]
      }
      frame "Configure App Image" {
        # "Update additional information (name, verison, description)\nstored with the selected application image"
        n270 = Unbundle By Name(w457) -> ("App Images Settings.App Images Temp Folder"=w453:path, "App Images Information"=w459:T13[])
        n271 = Decimal String To Number(string=w460) -> (number=w455:i32)  [unwired: 3 out]
        n272 = Index Array(array=w459, index=w455) -> (element=w454:T13)
        n273 = call "rad_Configure Application Image.vi"("Temp Folder"=w453, "error in (no error)"=w452, "App Images Information"=w454) -> ("error out"=w449:errorcluster, "Cancelled"=w447:bool, "App Images Information"=w448:T13)  [unwired: 6 in]
        n274 = Replace Array Subset(array=w459, new element=w448, index=w455) -> (w458:T13[])
        n275 = case shown="False" w447 {
          tunnel: [w464 w465] -> w451
          tunnel: w450 -> [w462 _]
          tunnel: w449 -> [w461 w465]
          frame False {
            n276 = call "Enqueue Message with Data.vi"("error in (no error)"=w461, "message ID"="Refresh AppImages", "queue in"=w462) -> ("error out"=w464:errorcluster)  [unwired: 7 in, 1 out]
          }
          frame True {
          }
        }
        n277 = Bundle By Name(cluster=w457, "App Images Information"=w458) -> (w456:T8)
      }
      frame "Configure AppImages Settings" {
        # "Update the selection of the folder where application images are stored"
        n278 = Unbundle By Name(w470) -> ("App Images Settings"=w469:T12)
        n279 = call "rad_Configure App Images Settings Dialog.vi"("App Images Settings"=w469) -> ("Cancelled"=w466:bool, "App Images Settings"=w468:T12)  [unwired: 1 in, 8 out]
        n280 = case shown="False" w466 {
          tunnel: w473 -> [w477 _]
          tunnel: w472 -> [w475 w478]
          tunnel: [w474 w478] -> w467
          frame False {
            n281 = call "Enqueue Message with Data.vi"("error in (no error)"=w475, "message ID"="Refresh AppImages", "queue in"=w477) -> ("error out"=w474:errorcluster)  [unwired: 7 in, 1 out]
          }
          frame True {
          }
        }
        n282 = Bundle By Name(cluster=w470, "App Images Settings"=w468) -> (w471:T8)
      }
      frame "View App Image Info" {
        n283 = Unbundle By Name(w483) -> ("App Images Information"=w482:T13[])
        n284 = Decimal String To Number(string=w480) -> (number=w479:i32)  [unwired: 2 in, 1 out]
        n285 = Index Array(array=w482, index=w479) -> (element=w481:T13)
        n286 = call "rad_View App Image Info.vi"("App Images Information"=w481) -> ()  [unwired: 11 in]
      }
      frame "Compare App Image" {
        n287 = Scan From String(format string="%[^(]", input string=w487) -> (remaining string=w486:string, output 1=w488:string)  [unwired: 2 in, 3 out]
        n288 = case shown="\"Image Target Compare\"" w488 {
          tunnel: w491 -> [w503 w532 w538]
          tunnel: w490 -> [w500 w524 w543]
          tunnel: w486 -> [w502 w534 _]
          tunnel: [w495 w522 w542] -> w485
          frame "Image Target Compare" {
            n289 = Unbundle By Name(w503) -> ("App Images Settings.App Images Folder"=w494:path, "App Images Settings.App Images Temp Folder"=w498:path, "App Images Information"=w508:T13[], "Targets Information"=w504:T10[], "Filtered Targets"=w505:i32[])
            n290 = Scan From String(format string="(%[^)]):%d", input string=w502, error in=w500) -> (error out=w496:errorcluster, output 1=w507:string, output 2=w509:i32)  [unwired: 1 in, 4 out]
            n291 = while {
              shift-right: [w517] -> _
              shift-left: w507 -> [w519]
              tunnel: w505 -> [w514]
              tunnel: w504 -> [w512]
              tunnel: [w511] -> w501 mode=indexing
              stop <- w516 stop-if-true
              n292 = Scan From String(format string="%d,", input string=w519) -> (remaining string=w517:string, output 1=w513:i32)  [unwired: 2 in, 3 out]
              n293 = Index Array(array=w514, index=w513) -> (element=w515:i32)
              n294 = Empty String/Path?(string/path=w517) -> (empty?=w516:bool)
              n295 = Index Array(array=w512, index=w515) -> (element=w511:T10)
            }
            n296 = Index Array(array=w508, index=w509) -> (element=w506:T13)
            n297 = Index Array(array=w501) -> (element=w492:T10)  [unwired: 1 in]
            n298 = Unbundle By Name(w506) -> ("AppImage Path"=w499:path)
            n299 = call "rad_RT Image Compare Dialog.vi"("App Images Repository"=w494, "Begin Automatically? (F)"=TRUE ("Show Front Panel?"), "Temp Folder"=w498, "error in (no error)"=w496, "Operation"=rad_Comparison_Modes."Compare Local Image With Controller", "Target settings"=w492, "Original Image Path"=w499) -> ("error out"=w495:errorcluster)  [unwired: 4 in]
          }
          frame "Only Image Selected" {
            n300 = Unbundle By Name(w532) -> ("App Images Settings.App Images Folder"=w521:path, "App Images Settings.App Images Temp Folder"=w527:path, "App Images Information"=w531:T13[])
            n301 = Scan From String(format string="(%d", input string=w534, error in=w524) -> (error out=w523:errorcluster, output 1=w530:i32)  [unwired: 1 in, 3 out]
            n302 = Index Array(array=w531, index=w530) -> (element=w529:T13)
            n303 = Unbundle By Name(w529) -> ("AppImage Path"=w528:path)
            n304 = call "rad_RT Image Compare Dialog.vi"("App Images Repository"=w521, "Begin Automatically? (F)"=FALSE ("Operate Headlessly?"), "Temp Folder"=w527, "error in (no error)"=w523, "Operation"=rad_Comparison_Modes."Compare Local Image With Controller", "Target settings"=T10 {"Hostname"="", "Serial number"="", "Product name"="", "Product code"=0, "System status"="", "Credential type"=enum."None/Unlocked", "User added?"=FALSE, "Primary NIC"={"MAC address"="", "IP Address Request Mode"=0, "IP address"="", "Subnet mask"="", "Gateway"="", "DNS server"=""}}, "Original Image Path"=w528) -> ("error out"=w522:errorcluster)  [unwired: 4 in]
          }
          frame "Generic Compare", Default {
            n305 = Unbundle By Name(w538) -> ("App Images Settings.App Images Folder"=w536:path, "App Images Settings.App Images Temp Folder"=w537:path)
            n306 = call "rad_RT Image Compare Dialog.vi"("App Images Repository"=w536, "Begin Automatically? (F)"=FALSE ("Operate Headlessly?"), "Temp Folder"=w537, "error in (no error)"=w543, "Operation"=rad_Comparison_Modes."Compare Local Image With Controller", "Target settings"=T10 {"Hostname"="", "Serial number"="", "Product name"="", "Product code"=0, "System status"="", "Credential type"=enum."None/Unlocked", "User added?"=FALSE, "Primary NIC"={"MAC address"="", "IP Address Request Mode"=0, "IP address"="", "Subnet mask"="", "Gateway"="", "DNS server"=""}}, "Original Image Path"=path "") -> ("error out"=w542:errorcluster)  [unwired: 4 in]
          }
        }
      }
      frame "Delete App Image" {
        n307 = Unbundle By Name(w560) -> ("App Images Information"=w559:T13[])
        n308 = Decimal String To Number(string=w558) -> (number=w557:i32)  [unwired: 2 in, 1 out]
        n309 = Index Array(array=w559, index=w557) -> (element=w556:T13)
        n310 = Unbundle By Name(w556) -> ("AppImage Path"=w551:path, "AppImage Properties.Name"=w553:string, "AppImage Properties.Version"=w544:string)
        n311 = Concatenate Strings("Are you sure you want to delete " ("string"), w553, " version " ("string"), w544, "?" ("string")) -> (w552:string)
        n312 = Two Button Dialog(message=w552, 2:"Delete" ("button name (\"OK\")")) -> (T button?=w550:bool)  [unwired: 1 in]
        n313 = case shown="True" w550 {
          tunnel: w551 -> [_ w567]
          tunnel: w549 -> [w561 w566]
          tunnel: [w561 w564] -> w548
          tunnel: w547 -> [_ w563]
          frame False {
          }
          frame True {
            n314 = Delete(path (use dialog)=w567, error in=w566) -> (error out=w565:errorcluster)  [unwired: 3 in, 2 out]
            n315 = call "Enqueue Message with Data.vi"("error in (no error)"=w565, "message ID"="Refresh AppImages" ("Message Name"), "queue in"=w563) -> ("error out"=w564:errorcluster)  [unwired: 7 in, 1 out]
          }
        }
      }
      frame "Retrieve AppImage" {
        # "Retrieve the application image\nfrom the selected RT target."
        n316 = Unbundle By Name(w576) -> ("App Images Settings.App Images Temp Folder"=w578:path, "App Images Settings.App Images Folder"=w572:path, "Targets Information"=w568:T10[], "Filtered Targets"=w569:i32[])
        n317 = Decimal String To Number(string=w584) -> (number=w583:i32)  [unwired: 3 out]
        n318 = Index Array(array=w569, index=w583) -> (element=w585:i32)
        n319 = Index Array(array=w568, index=w585) -> (element=w570:T10)
        n320 = call "rad_Retrieve Application Image From Target.vi"("App Images Temp Folder"=w578, "error in (no error)"=w582, "Target settings"=w570, "App Images Folder"=w572) -> ("error out"=w581:errorcluster, "Cancelled"=w573:bool, "New App Image Path"=w577:path)  [unwired: 3 in, 2 out]
        n321 = Strip Path(path=w577) -> (stripped path=w574:path)  [unwired: 1 out]
        n322 = case shown="False" w573 {
          tunnel: w581 -> [w589 w590]
          tunnel: [w588 w590] -> w580
          tunnel: w579 -> [w587 _]
          frame False {
            n323 = call "Enqueue Message with Data.vi"("error in (no error)"=w589, "message ID"="Refresh AppImages" ("Message Name"), "queue in"=w587) -> ("error out"=w588:errorcluster)  [unwired: 7 in, 1 out]
          }
          frame True {
          }
        }
        n324 = Select(t=w572, s=w573, f=w574) -> (s? t:f=w571:path)
        n325 = Bundle By Name(cluster=w576, "App Images Settings.App Images Folder"=w571) -> (w575:T8)
      }
      frame "Deploy AppImage" {
        # "Deploy the selected application image to the select RT target(s)"
        n326 = Unbundle By Name(w607) -> ("App Images Settings.App Images Temp Folder"=w597:path, "App Images Information"=w603:T13[], "Targets Information"=w599:T10[], "Filtered Targets"=w600:i32[])
        n327 = Scan From String(format string="(%[^)]):%d", input string=w606) -> (output 1=w602:string, output 2=w604:i32)  [unwired: 2 in, 5 out]
        n328 = while {
          shift-right: [w619] -> _
          shift-left: w602 -> [w621]
          tunnel: w600 -> [w616]
          tunnel: w599 -> [w614]
          tunnel: [w613] -> w596 mode=indexing
          stop <- w618 stop-if-true
          n329 = Scan From String(format string="%d,", input string=w621) -> (remaining string=w619:string, output 1=w615:i32)  [unwired: 2 in, 3 out]
          n330 = Index Array(array=w616, index=w615) -> (element=w617:i32)
          n331 = Empty String/Path?(string/path=w619) -> (empty?=w618:bool)
          n332 = Index Array(array=w614, index=w617) -> (element=w613:T10)
        }
        n333 = Index Array(array=w603, index=w604) -> (element=w601:T13)
        n334 = Unbundle By Name(w601) -> ("AppImage Path"=w598:path)
        n335 = call "rad_Deploy Application Image.vi"("App Image Temp Folder"=w597, "error in (no error)"=w595, "Selected Targets"=w596, "App Image Path"=w598) -> ("error out"=w593:errorcluster, "Cancelled"=w591:bool)  [unwired: 6 out]
        n336 = case shown="False" w591 {
          tunnel: [w611 w612] -> w594
          tunnel: w593 -> [w610 w612]
          tunnel: w592 -> [w608 _]
          frame False {
            n337 = call "Enqueue Message with Data.vi"("error in (no error)"=w610, "message ID"="Refresh Targets" ("Message Name"), "queue in"=w608) -> ("error out"=w611:errorcluster)  [unwired: 7 in, 1 out]
          }
          frame True {
          }
        }
      }
      frame "Convert Images" {
        n338 = Unbundle By Name(w623) -> ("App Images Settings.App Images Folder"=w622:path)
        n339 = call "Util_ConvertImageToLatest.vi"("error in (no error)"=w628, "Image Path"=w622) -> ("error out"=w626:errorcluster)  [unwired: 9 in]
        n340 = call "Enqueue Message with Data.vi"("error in (no error)"=w626, "message ID"="Refresh AppImages" ("Message Name"), "queue in"=w624) -> ("error out"=w625:errorcluster)  [unwired: 7 in, 1 out]
      }
    }
    n341 = local write "State"(w167) -> ()
  }
  n342 = call "Resize Front Panel Main.vi"("Left Listbox"=w29, "Top Level VI"=w30, "Stop"=w31, "Number of Columns"=4, "Right Listbox"=w28, "Left Splitter"=w27, "Right Splitter"=w26, "Left Pane Items"=w20, "Mid Pane Items"=w16, "Right Pane Items"=w11) -> ()  [unwired: 5 in, 1 out]
  n343 = local write "Exit"(w10) -> ()
